vi "MultipleMeasurements_XcpDiffId.vi"() -> ()   [LabVIEW 2019]
doc: "This VI serves as a basic example how to set up a measurement task with several channels.\n\nSelect an A2L data base and a set of measurement channels from it and run the VI. It will display all measurements defined in the chart window. Click Stop when you are done."
uses:
  DAQList/DAQList.lvclass/DAQList.ctl
  A2L_Utility/Private/Find CAN_ID.vi
  DAQList/XcpCommand/SendCommands.vi
  DAQList/DatabaseGeneration/CreateCluster.vi
  DAQList/DatabaseGeneration/CreateFrames.vi
  DAQList/XnetRead/InitXnet.vi
  DAQList/DatabaseGeneration/CreateSignals.vi
  DAQList/DatabaseGeneration/CreateSignals_SingleByte.vi
  DAQList/XnetRead/ProcessMeaSplit.vi
  A2L_Utility/Private/ParseNumeric.vi
  DAQList/XnetRead/InitMeaSplitInfo2.vi
  DAQList/DatabaseGeneration/SubVI_SetMeasProp.vi
  DAQList/DatabaseGeneration/SubVI_ProcessMeasName.vi
  DAQList/XnetRead/SubVI_MergeData2.vi
  <vilib>/ECUMC/ECUMC.llb/MC Get Property.vi
  <vilib>/ECUMC/ECUMC.llb/MC Get Prop DB File Name.vi
  <vilib>/Utility/file.llb/Read Delimited Spreadsheet.vi
  <vilib>/Utility/file.llb/Read Delimited Spreadsheet (string).vi
  <vilib>/Utility/error.llb/Error Cluster From Error Code.vi
  <vilib>/xnet/xnet.llb/XNET Create Session.vi
  <vilib>/xnet/xnet.llb/XNET Create Session (Frame Input Stream).vi
  <vilib>/xnet/xnet.llb/XNET Start.vi
  <vilib>/ECUMC/ECUMC.llb/MC DAQ List Initialize.vi
  <vilib>/ECUMC/ECUMC.llb/MC ECU Connect.vi
  <vilib>/ECUMC/ECUMC.llb/MC DAQ Start Stop.vi
  <vilib>/xnet/xnet.llb/XNET Read.vi
  <vilib>/xnet/xnet.llb/XNET Read (Frame CAN).vi
  <vilib>/xnet/xnet.llb/XNET Clear.vi
  DAQList/XcpCommand/FilterCommands.vi
  <vilib>/ECUMC/ECUMC.llb/MC Get Prop XCP CAN IO Mode.vi
  <vilib>/ECUMC/ECUMC.llb/MC Get Prop XCP Baud Rate 64.vi
  <vilib>/ECUMC/ECUMC.llb/MC Get Prop XCP FD Baud Rate 64.vi
  <vilib>/xnet/xnet.llb/XNET Database Create Object.vi
  <vilib>/xnet/xnet.llb/XNET Database Create (Cluster).vi
  <vilib>/xnet/xnet.llb/XNET Database Create (Frame).vi
  <vilib>/Utility/file.llb/Application Directory.vi
  <vilib>/xnet/xnet.llb/XNET Database Save.vi
  <vilib>/ECUMC/ECUMC.llb/MC Get Prop Meas Address.vi
  <vilib>/xnet/xnet.llb/XNET Database Create (Signal).vi
  <vilib>/xnet/xnet.llb/XNET Database Create (Subframe).vi
  <vilib>/ECUMC/ECUMC.llb/MC Get Prop Meas Data Type.vi
  DAQList/TypeDef/Global.vi
  <vilib>/xnet/xnet.llb/XNET Database Create (Dynamic Signal).vi
  <vilib>/ECUMC/ECUMC.llb/MC Get Prop Meas Comment.vi
  <vilib>/ECUMC/ECUMC.llb/MC Get Prop Meas Scaling Offset.vi
  <vilib>/ECUMC/ECUMC.llb/MC Get Prop Meas Scaling Factor.vi
  <vilib>/ECUMC/ECUMC.llb/MC Get Prop Meas Minimum.vi
  <vilib>/ECUMC/ECUMC.llb/MC Get Prop Meas Maximum.vi
  <vilib>/ECUMC/ECUMC.llb/MC Get Prop Meas Byte Order.vi
  <vilib>/ECUMC/ECUMC.llb/MC Get Prop Meas Unit.vi
  <vilib>/xnet/xnet.llb/XNET Create Session (Signal Input Waveform).vi
  <vilib>/xnet/xnet.llb/XNET Read (Signal Waveform) .vi
  <vilib>/xnet/xnet.llb/XNET Stop.vi
  <vilib>/ECUMC/ECUMC.llb/MC DAQ Clear.vi
  DAQList/DAQList.lvclass
  <vilib>/ECUMC/ECUMC.lvlib
  A2L Utility.lvlib
panel:
  in  "ID Source":bool
  in  "ID Type":bool
  in  "Number of DAQ List":i32=8
  in  "DTO_ID":u32 format="%.0x"
  in  "Measurement List":string[](array[string])=["OneDimTimeSig", "PWM_Signal", "Sinus1", "Sinus2"]
  in  "CAN Interface":refnum<k21>="CAN1"
  in  "Stop":bool
  out "Measurements":waveform(dbl)[](graph)
  in  "A2L Database":path
  # "DISCLAIMER: The attached Code is provided As Is. It has not been tested or validated as a product, for use in a deployed application or system, or for use in hazardous environments. You assume all risks for use of the Code and use of the Code is subject to the Sample Code License Terms which can be found at: http://ni.com/samplecodelicense\n\nImportant Note \n1. This example only works with XCP_ON_CAN.\n2. This example does not work if the DAQ List ID is similar with DTO_ID thus does not work with XCP Demo ECU.\n3. This example does not support dynamic DAQ lists and does not take event channel into consideration."
  # "A2L Database and Connection"
  # "Measurements"
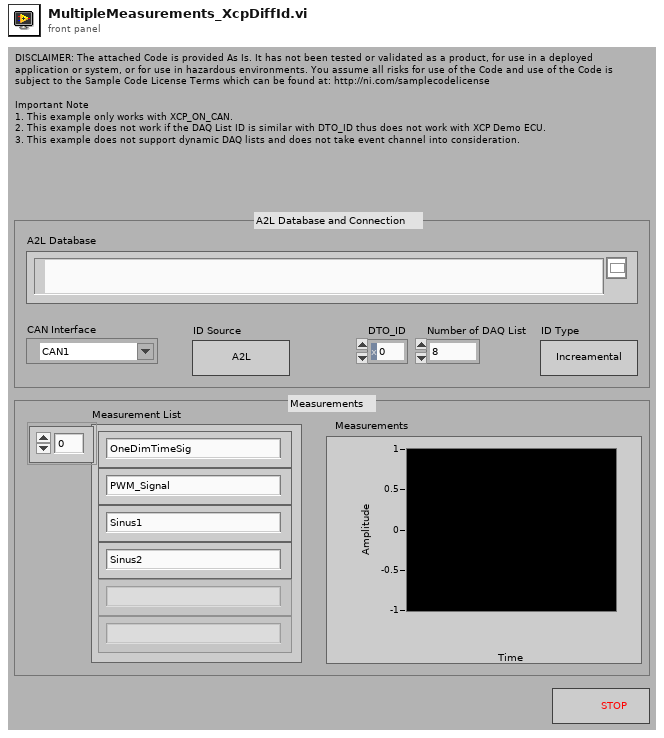
[diagram p1: front panel]
types:
  T1 = typedef "ECUMC.lvlib/MC Reference.ctt" = u32
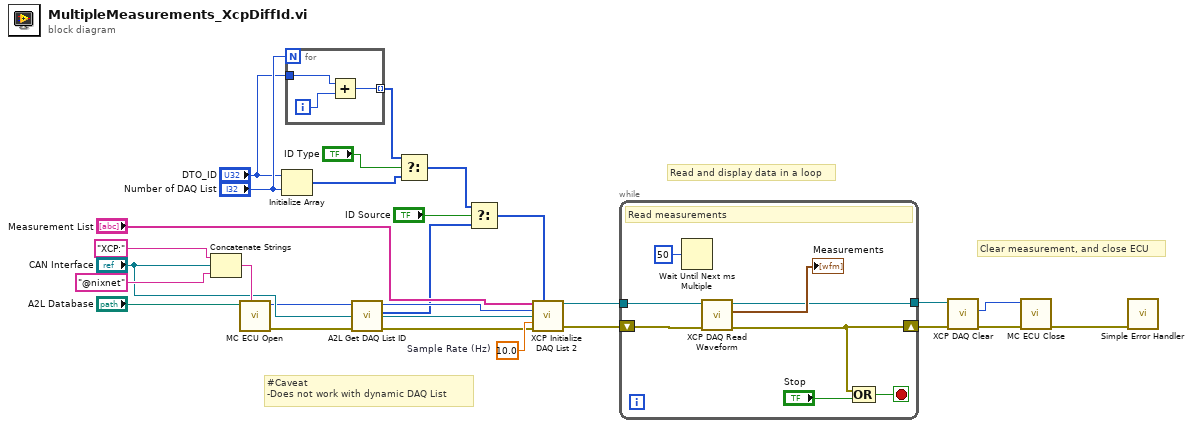
[diagram p0: block diagram]
diagram:
  w9 = 10.0  # Sample Rate (Hz)
  # "Clear measurement, and close ECU"
  # "Read and display data in a loop"
  # "#Caveat\n-Does not work with dynamic DAQ List"
  n1 = Concatenate Strings("XCP:" ("string"), "CAN Interface", "@nixnet" ("string")) -> (w26:string)
  n2 = call <vilib>:"MC ECU Open.vi"("protocol and interface"=w26, "DB path"="A2L Database") -> ("error out"=w4:errorcluster, "ECU ref out"=w7:T1)  [unwired: 1 in, 7 out]
  n3 = Initialize Array("DTO_ID", "Number of DAQ List") -> (w21:u32[])
  n4 = for {
    N: "Number of DAQ List" -> [_]
    tunnel: "DTO_ID" -> [w30]
    tunnel: [w28] -> w18 mode=indexing
    i -> [w29]
    n5 = Add(x=w30, y=w29) -> (x+y=w28:u32)
  }
  n6 = call "A2L Get DAQ List ID.vi"("error in (no error)"=w4, "ECU ref in"=w7) -> ("error out"=w5:errorcluster, "DAQ List IDs"=w1:u32[], "ECU ref out"=w6:T1)  [unwired: 7 in]
  n7 = Select(t=w18, s="ID Type", f=w21) -> (s? t:f=w3:u32[])
  n8 = Select(t=w3, s="ID Source", f=w1) -> (s? t:f=w2:u32[])
  n9 = call "XCP Initialize DAQ List 2.vi"("Measurement List"="Measurement List", "DTO IDs"=w2, "ECU ref in"=w6, "CAN Interface"="CAN Interface", "Sample Rate (Hz)"=w9, "error in (no error)"=w5) -> ("DAQList out"=w12:refnum<class "DAQList.lvclass">, "error out"=w11:errorcluster)  [unwired: 8 in]
  n10 = while {
    shift-right: [w33] -> w16
    shift-left: w11 -> [w34]
    tunnel: [w32] -> w13
    tunnel: w12 -> [w31]
    stop <- w38 stop-if-true
    # "Read measurements"
    n11 = Wait Until Next ms Multiple(millisecond multiple=u32 50) -> ()  [unwired: 1 out]
    n12 = call "XCP DAQ Read Waveform.vi"("error in (no error)"=w34, "DAQList in"=w31) -> ("error out"=w33:errorcluster, "Data"=→"Measurements":waveform(dbl)[], "DAQList out"=w32:refnum<class "DAQList.lvclass">)  [unwired: 7 in]
    n13 = Compound Arithmetic op=OR(w33, "Stop") -> (w38:bool)
  }
  n14 = call "XCP DAQ Clear.vi"("error in (no error)"=w16, "DAQList in"=w13) -> ("error out"=w15:errorcluster, "ECU ref out"=w14:T1)  [unwired: 8 in]
  n15 = call <vilib>:"MC ECU Close.vi"("error in"=w15, "ECU ref in"=w14) -> ("error out"=w23:errorcluster)  [unwired: 9 out]
  n16 = call <vilib>:"Simple Error Handler.vi"("error in (no error)"=w23) -> ()  [unwired: 1 in, 8 out]
